vi "AlazarFFTGetMaxTriggerRepeatRate.vi"(4 "error in (no error)":errorcluster, 6 "FFT Size":u32, 7 "DSP Handle":u64) -> (0 "error out":errorcluster, 1 "Return Code":u32, 2 "Trigger Repeat Rate":dbl, 3 "DSP Handle 2":u64)   [LabVIEW 2018]
doc: "Get the total number of board systems detected."
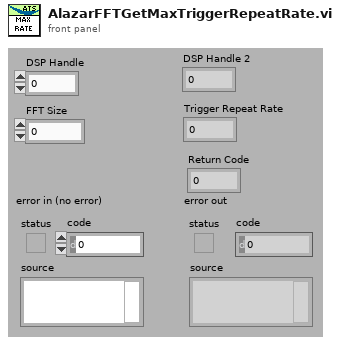
[diagram p1: front panel]
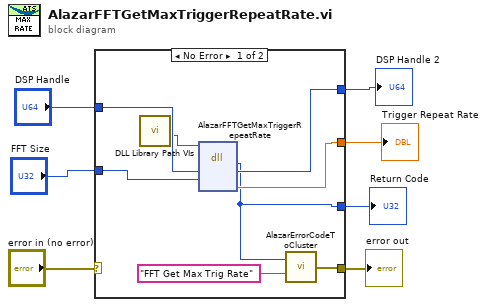
[diagram p0: block diagram]
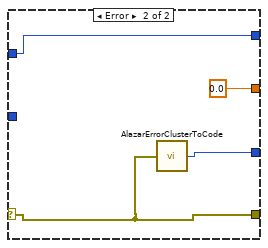
[diagram p2: hidden frame]
diagram:
  n1 = case shown="No Error" "error in (no error)" {
    selector: "error in (no error)" -> [_ w19]
    tunnel: [w11 w19] -> w6
    tunnel: "FFT Size" -> [w15 _]
    tunnel: "DSP Handle" -> [w14 w16]
    tunnel: [w13 w16] -> w3
    tunnel: [w9 w18] -> w2
    tunnel: [w10 0.0] -> w1
    frame No Error {
      n2 = call "DLL Library Path VIs.vi"() -> ("Alazar"=w8:path)  [unwired: 9 in, 2 out]
      n3 = dll-call lib="C:/Project/SerialSectOCT - FFT GPU/SerialSectOCT/Labview Software/DLL/ATSApi.dll" fn="AlazarFFTGetMaxTriggerRepeatRate"(path in=w8, "handle"=w14, "fft_size"=w15) -> ("return type"=w9:u32, "handle"=w13:u64, "rate"=w10:dbl)  [unwired: 4 in, 2 out]
      n4 = call "AlazarErrorCodeToCluster.vi"("Message"="FFT Get Max Trig Rate", "Error Code"=w9) -> ("error out"=w11:errorcluster)
    }
    frame Error {
      n5 = call "AlazarErrorClusterToCode.vi"("error in (no error)"=w19) -> ("Error Code"=w18:u32)
    }
  }
  "error out" <- w6
  "Trigger Repeat Rate" <- w1
  "DSP Handle 2" <- w3
  "Return Code" <- w2
